vi "Blank Bits.vi"(2 "Blanking Bits":u8 format="%.0b", 7 "Expected Input":u8 format="%.0b", 11 "Readback Value":u8 format="%.0b") -> (8 "Output":u8 format="%.0b", 15 "Equal?":bool)   [LabVIEW 2010]
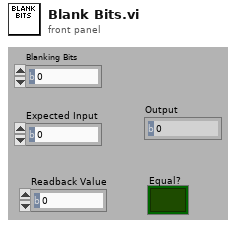
[diagram p1: front panel]
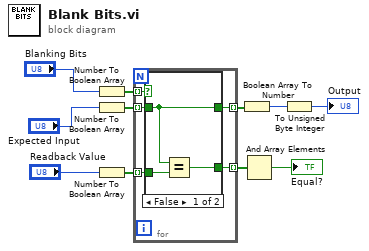
[diagram p0: block diagram]
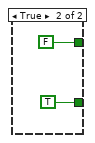
[diagram p2: hidden frame]
diagram:
  n1 = Number To Boolean Array(number="Blanking Bits") -> (Boolean array=w7:bool[])
  n2 = Number To Boolean Array(number="Expected Input") -> (Boolean array=w6:bool[])
  n3 = Number To Boolean Array(number="Readback Value") -> (Boolean array=w3:bool[])
  n4 = for {
    tunnel: w7 -> [w16] mode=indexing
    tunnel: w6 -> [w15] mode=indexing
    tunnel: [w14] -> w10 mode=indexing
    tunnel: w3 -> [w13] mode=indexing
    tunnel: [w12] -> w2 mode=indexing
    n5 = case shown="False" w16 {
      tunnel: w15 -> [w18 _]
      tunnel: [w18 FALSE] -> w14
      tunnel: w13 -> [w19 _]
      tunnel: [w17 TRUE] -> w12
      frame False {
        n6 = Equal?(x=w18, y=w19) -> (x = y?=w17:bool)
      }
      frame True {
      }
    }
  }
  n7 = Boolean Array To Number(Boolean array=w10) -> (number=w11:u32)
  n8 = And Array Elements(Boolean array=w2) -> (logical AND=→"Equal?":bool)
  n9 = To Unsigned Byte Integer(number=w11) -> (unsigned 8bit integer=→"Output":u8)
